vi "harp convert to csv.vi"() -> ()   [LabVIEW 2010]
uses:
  <vilib>/Utility/sysdir.llb/System Directory Type.ctl
panel:
  in  "error":string
  in  "don't\nask":bool
  in  "dummy 2":dbl caption="Available hidden commands:\nbootloader\ncreatecode\nresetcounters\nhardware"
  in  "ShowList":bool
  out "CameraBitPosition":i32
  out "Files to convert to CSV: 2":string
  in  "Match pattern: 2":string
  in  "Include subfolders: 2":bool=TRUE
  out "Overall progress: 2":dbl(slide) scale=0.0..1.0
  in  "Path (folder) 2":path caption="Path"
  out "Binary Harp folder: 2":string
  out "File progress: 2":dbl(slide) scale=0.0..1.0
  in  "Overwrite .csv files: 2":bool=TRUE
  in  "File extension: 2":string=".bin"
  in  "Execute parse on computer's RAM (faster): 2":bool=TRUE
  in  "System 2":bool
  in  "Create \"read me\" information file: 2":bool=TRUE
  in  "Filter: 2":T1(ring)
  in  "List: 2":string
  in  "Read 2":bool=TRUE
  in  "Write 2":bool=TRUE
  in  "Event 2":bool=TRUE
  in  "Save only if no error: 2":bool=TRUE
  in  "Round time to 4th decimal place: 2":bool=TRUE
  in  "Include entire information: 2":bool
  in  "Insert Bit Demux Elements at the end: 2":bool
  in  "For separation, use Tab instead of Comma:":bool
  out "System (copy)":bool
  in  "abort":bool
  out "conversion\ntime":u32
  in  "dummy":dbl
  out "Error Ctrl":bool
  in  "Create file with metadata information:":bool=TRUE
  in  "Show options":bool
  in  "Tab Control":T2(tab)
  in  "Tips":bool
  in  "Path (file)":path caption="Path"
  out "(1) Binary Harp file:":string
  in  "Convert":bool
  out "Progress:":dbl(slide) scale=0.0..1.0
  in  "Tips":bool
  out "Files to convert to CSV:":string="\r\n"
  in  "(14) Match pattern:":string
  in  "(12) Include subfolders:":bool=TRUE
  out "Overall progress:":dbl(slide) scale=0.0..1.0
  in  "Path (folder)":path caption="Path"
  out "(10) Binary Harp folder:":string
  in  "Convert 2":bool
  out "File progress:":dbl(slide) scale=0.0..1.0
  in  "(11) Overwrite .csv files:":bool=TRUE
  in  "(13) File extension:":string=".bin"
  in  "(41) Execute parse on computer's RAM (faster):":bool
  in  "System":bool
  in  "(30) Create \"read me\" information file:":bool=TRUE
  in  "(39) Filter:":T3(ring)
  in  "(40) List:":string caption="Separate the registers with a comma.\nExample: 8,32,33"
  in  "(32) Read":bool
  in  "(33) Write":bool
  in  "(34) Event":bool=TRUE
  in  "(35) Save only if no error:":bool=TRUE
  in  "(36) Round time to 4th decimal place:":bool=TRUE
  in  "(38) Include entire information:":bool
  in  "(37) Insert Bit Demux Elements at the end:":bool
  in  "Add register":bool
  in  "Quit":bool
  in  "Minimize":bool
  in  "Cam Tip":bool
  in  "Progress:":dbl(slide) scale=0.0..1.1
  in  "Convert 3":bool
  out "(60) Binary Harp file:":string
  in  "harp .bin":path caption="Path"
  out "(61) Camera metadata .csv file :":string
  in  "cam .csv":path caption="Path"
  in  "(62) Use Harp converted .csv file\nto timestamp the file:":bool=TRUE
  in  "Select Register":bool
  out "Pin name on the board:":string
  out "Raw Register Name:":string
  out "(64) Register Address:":i32
  in  "(63) Camera brand:":u16(ring) items=["PointGrey"]
  in  "EnableList":T4={"Cmd"=TRUE, "RegAdd"=TRUE, "Port"=FALSE, "Rsvd"=FALSE, "UTC"=TRUE, "Error"=FALSE, "Type"=FALSE, "NElements"=FALSE, "BitElementsColumn"=FALSE, "BitElementsAtTheEnd"=FALSE, "Read"=FALSE, "Write"=FALSE, "Event"=TRUE, "No Errors"=TRUE}
  # "Convert to CSV v1.9.0\nHardware Platform"
  # "Fractional number separation:"
  # "Separate the registers with a comma.\nExample: 8,32,33"
  # "Commands:"
  # "New columns will be added to the file\n(Port, Reserved, Error, Type and NumberOfElements)."
  # "The files with this pattern on the\nfile name will be converted to CSV.\nYou can leave it blank to select\nall files."
  # "Select the Harp binary file:"
  # "Select the folder where the Harp binary files exist:"
  # "The files with this pattern on the\nfile name will be converted to CSV.\nYou can leave it blank to select\nall files."
  # "Configuration of output files:"
  # "(31) Fractional number separation:"
  # "Commands:"
  # "New columns will be added to the file\n(Port, Reserved, Error, Type and NumberOfElements)."
  # "Select the files and the register:"
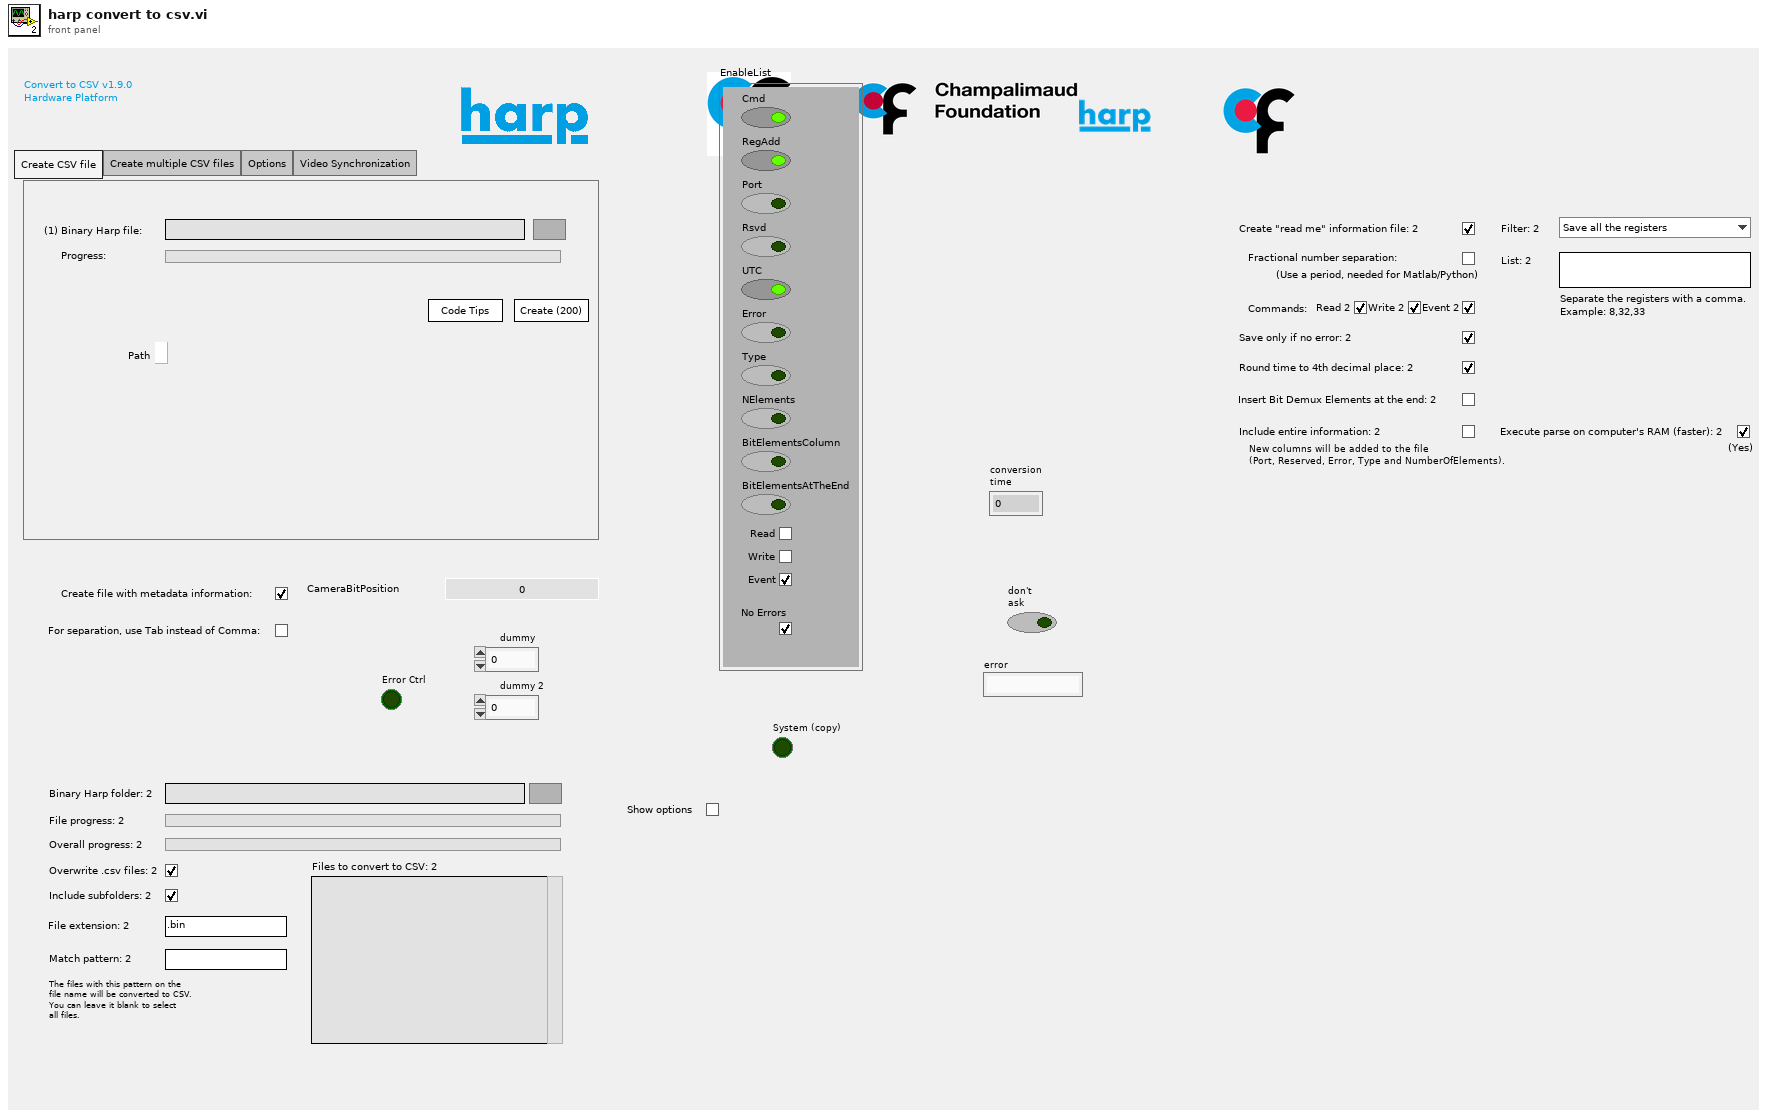
[diagram p1: front panel]
types:
  T1 = enum16{"Save all the registers", "Save only specific registers"}
  T2 = enum32{"Create CSV file", "Create multiple CSV files", "Options", "Video Synchronization"}
  T3 = enum16{"Save all the registers (0)", "Save only specific registers (1)"}
  T4 = cluster{"Cmd":bool, "RegAdd":bool, "Port":bool, "Rsvd":bool, "UTC":bool, "Error":bool, "Type":bool, "NElements":bool, "BitElementsColumn":bool, "BitElementsAtTheEnd":bool, "Read":bool, "Write":bool, "Event":bool, "No Errors":bool}
  T5 = enum32{"Invalid", "Standard", "Closed", "Hidden", "Minimized", "Maximized"}
  T6 = enum16{"Reset", "Get command", "Open files", "Freeze", "Unfreeze"}
  T7 = typedef "System Directory Type.ctl" = i32
  T8 = enum16{"open", "replace", "create", "open or create", "replace or create", "replace or create with confirmation"}
  T9 = enum32{"Create CSV file", "Create multiple CSV files", "Options"}
  T10 = enum8{"Enabled", "Disabled", "Disabled and Grayed Out"}
  T11 = cluster{"Create \"read me\" information file:":bool, "Create \"read me\" information file:":bool, "Create \"read me\" information file:":bool, "Create \"read me\" information file:":bool, "Create \"read me\" information file:":bool, "Create \"read me\" information file:":bool, "Create \"read me\" information file:":bool, "Create \"read me\" information file:":bool, "Create \"read me\" information file:":bool, "Filter:":enum16{"Save all the registers (0)", "Save only specific registers (1)"}, "List:":string, "Create \"read me\" information file:":bool, "List:":string, "List:":string, "Create \"read me\" information file:":bool, "Create \"read me\" information file:":bool, "List:":string, "List:":string, "List:":string, "List:":string, "Create \"read me\" information file:":bool, "List:":string, "RegisterAddress":i32, "List:":string, "RegisterAddress":i32}
  T12 = enum16{"Reset", "Get command", "Open files", "Freeze", "Unfreeze", "Save error"}
  T13 = enum16{"CreateBuffer", "WriteBytes", "WriteByte", "AvailableMemory", "OccupiedMemory", "CheckBytes", "ReadBytes"}
  T14 = cluster{"Device":string, "RegisterName":string, "PinBoardName":string, "CameraBitPosition":i32, "RegisterDescription":string, "IsUsedForCamera":bool, "RegisterAddress":i32, "RegisterRawName":string, "RegisterByteSize":i32}
  T15 = cluster{"(30) Create \"read me\" information file:":bool, "System":bool, "(32) Read":bool, "(33) Write":bool, "(34) Event":bool, "(35) Save only if no error:":bool, "(36) Round time to 4th decimal place:":bool, "(37) Insert Bit Demux Elements at the end:":bool, "(38) Include entire information:":bool, "(39) Filter:":enum16{"Save all the registers (0)", "Save only specific registers (1)"}, "(40) List:":string, "(41) Execute parse on computer's RAM (faster):":bool, "(1) Binary Harp file:":string, "(10) Binary Harp folder:":string, "(11) Overwrite .csv files:":bool, "(12) Include subfolders:":bool, "(13) File extension:":string, "(14) Match pattern:":string, "(60) Binary Harp file:":string, "(61) Camera metadata .csv file :":string, "(62) Use Harp converted .csv file\nto timestamp the file:":bool, "Raw Register Name:":string, "(64) Register Address:":i32, "Pin name on the board:":string, "CameraBitPosition":i32}
  T16 = cluster{"Timestamp(us)":dbl, "Command":u8, "Error":bool, "Register Address":u8, "Port":u8, "Number of Elements":u8, "Type":u8, "I8":i8, "U8":u8, "U16":u16, "I16":i16, "U32":u32, "I32":i32, "U64":u64, "I64":i64, "Float":sgl, "U8[]":u8[], "I8[]":i8[], "U16[]":u16[], "I16[]":i16[], "U32[]":u32[], "I32[]":i32[], "U64[]":u64[], "I64[]":i64[], "Float[]":sgl[]}
  T17 = enum16{"Left Button", "Center Button", "Right Button", "Window Close"}
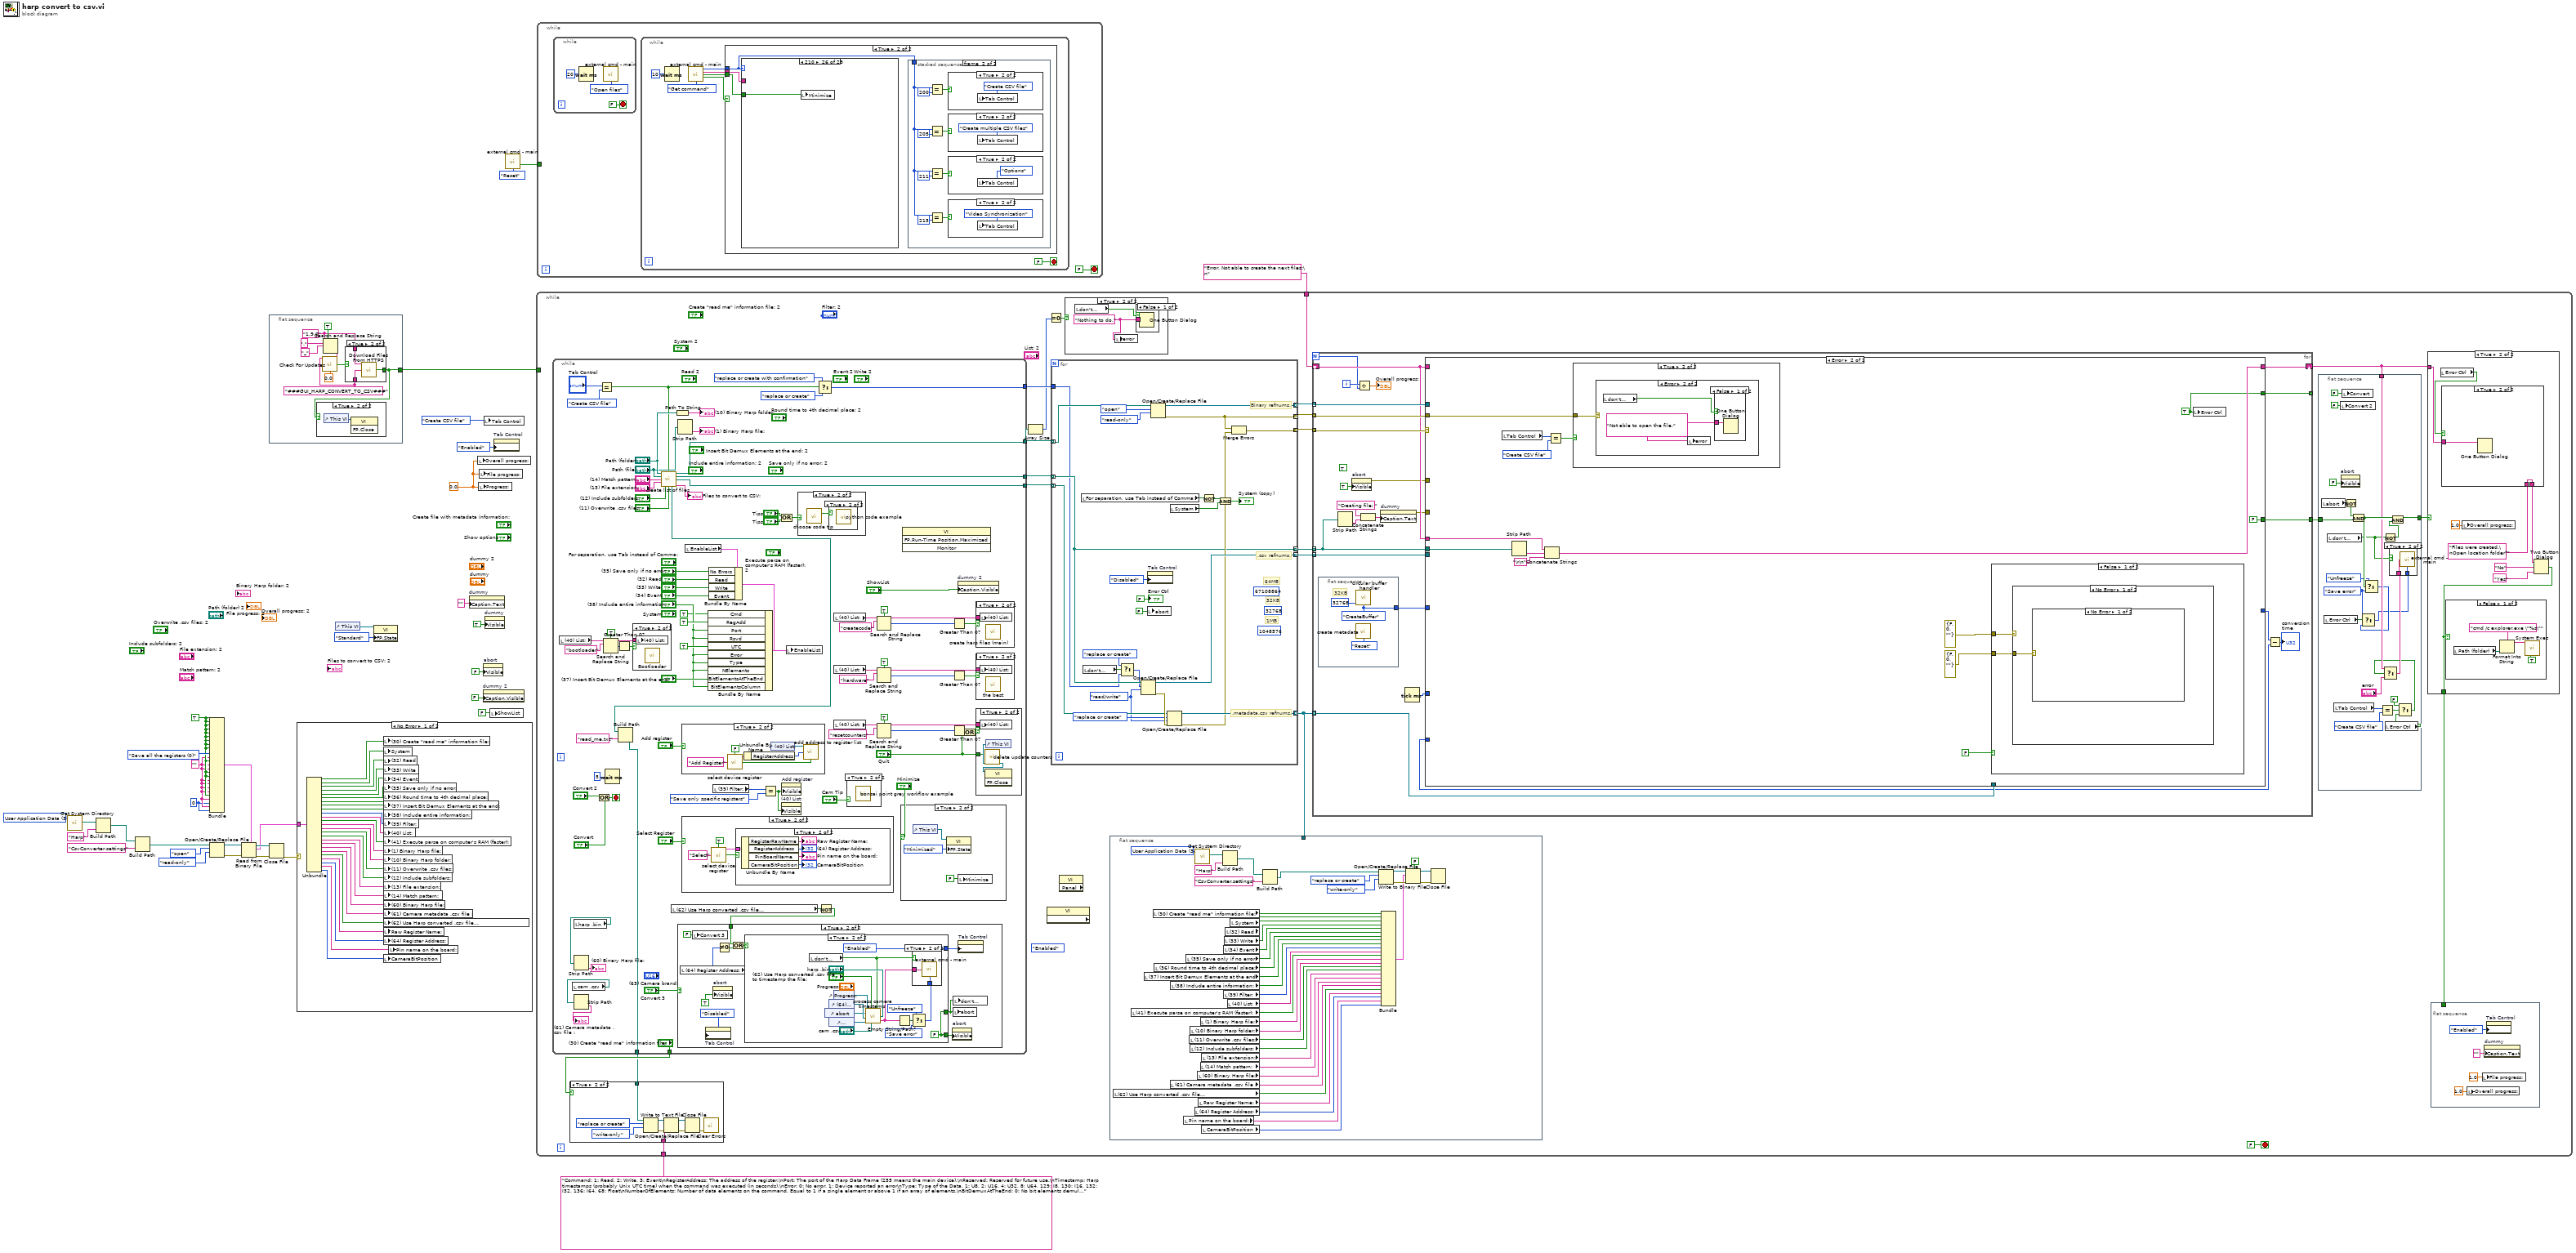
[diagram p0: block diagram]
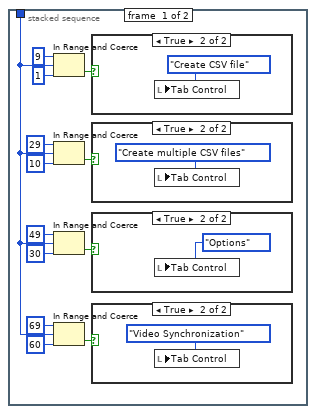
[diagram p3: hidden frame]
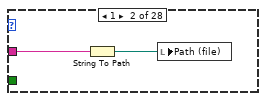
[diagram p13: hidden frame]
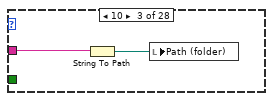
[diagram p14: hidden frame]
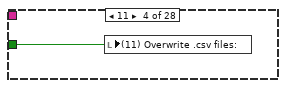
[diagram p15: hidden frame]
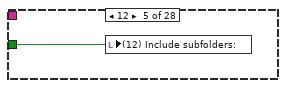
[diagram p16: hidden frame]
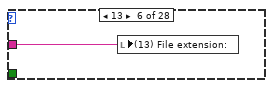
[diagram p17: hidden frame]
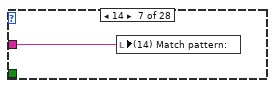
[diagram p18: hidden frame]
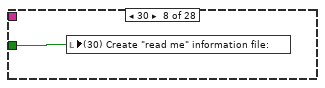
[diagram p19: hidden frame]
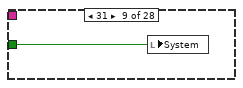
[diagram p20: hidden frame]
diagram:
  w6 = T7 3 items=["User Home"=0, "User Desktop"=1, "User Documents"=2, "User Application Data"=3, "User Preferences"=4, "User Temporary"=5, "Public Documents"=6, "Public Application Data"=7, "Public Preferences"=8, "Public Cache"=13, "System Core Libraries"=9, "System Installed Libraries"=10, "Application Files"=11, "Boot Volume Root"=12] ("system directory type")
  w9 = 0 ("RegisterAddress")
  w10 = "" ("List:")
  w11 = TRUE ("Create \"read me\" information file:")
  w32 = 0.0 ("Processing")
  n1 = call <vilib>:"Get System Directory.vi"("system directory type"=w6) -> ("system directory"=w7:path)  [unwired: 10 in]
  n2 = Build Path(base path=w7, name or relative path="Harp") -> (appended path=w5:path)
  n3 = Build Path(base path=w5, name or relative path="CsvConverter.settings") -> (appended path=w12:path)
  n4 = Bundle("Create \"read me\" information file:"=w11, "Create \"read me\" information file:"=w11, "Create \"read me\" information file:"=w11, "Create \"read me\" information file:"=w11, "Create \"read me\" information file:"=w11, "Create \"read me\" information file:"=w11, "Create \"read me\" information file:"=w11, "Create \"read me\" information file:"=w11, "Create \"read me\" information file:"=w11, "Filter:"=T3."Save all the registers (0)", "List:"=w10, "Create \"read me\" information file:"=w11, "List:"=w10, "List:"=w10, "Create \"read me\" information file:"=w11, "Create \"read me\" information file:"=w11, "List:"=w10, "List:"=w10, "List:"=w10, "List:"=w10, "Create \"read me\" information file:"=w11, "List:"=w10, "RegisterAddress"=w9, "List:"=w10, "RegisterAddress"=w9) -> (w19:T11)  [unwired: 1 in]
  n5 = Open/Create/Replace File(file path (use dialog)=w12, operation (0:open)=T8."open", access (0:read/write)=enum16{"read/write", "read-only", "write-only"}."read-only") -> (refnum out=w17:refnum<file>, error out=w16:errorcluster)  [unwired: 3 in, 1 out]
  n6 = Read from Binary File(5:w19, 8:w16, 11:w17) -> (0:w21:errorcluster, 2:w20:T11, 3:w22:refnum<file>)  [unwired: 3 in, 1 out]
  n7 = flat-sequence {
    tunnel: [w36] -> w26
    frame #0 {
      w39 = "1.9.0" ("current version")
      w38 = "###GUI_HARP_CONVERT_TO_CSV###" ("name or relative path")
      n8 = Search and Replace String(replace all?=TRUE ("replace all? (F)"), input string=w39, search string=".", replace string="_" ("replace string (\"\")")) -> (result string=w40:string)  [unwired: 4 in, 3 out]
      n9 = call "Check For Updates.vi"("GUI search key"=w38, "shortcut key"=w40, "timeout (days)"=0.0) -> ("check for updates"=w37:bool)  [unwired: 12 in]
      n10 = case shown="True" w37 {
        tunnel: w38 -> [_ w48]
        tunnel: w39 -> [_ w47]
        tunnel: [FALSE ("updated") w46] -> w36
        frame False {
        }
        frame True {
          n11 = call "Download Files From HTTPS.vi"("current version"=w47, "GUI search key"=w48) -> ("updated"=w46:bool)  [unwired: 13 in]
        }
      }
      n12 = case shown="True" w36 {
        frame False {
        }
        frame True {
          n13 = control-ref of="This VI"() -> (w44:refnum<vi>)
          n14 = invoke class="VI" method="FP.Close"(reference=w44) -> ()  [unwired: 2 in, 3 out]
        }
      }
    }
  }
  n15 = Close File(refnum=w22, error in=w21) -> (error out=w23:errorcluster)  [unwired: 1 out]
  n16 = case shown="No Error" w23 {
    tunnel: w20 -> [w74 _]
    frame No Error {
      n17 = Unbundle(w74) -> ("Create \"read me\" information file:"=w73:bool, "Create \"read me\" information file:"=w72:bool, "Create \"read me\" information file:"=w71:bool, "Create \"read me\" information file:"=w70:bool, "Create \"read me\" information file:"=w69:bool, "Create \"read me\" information file:"=w68:bool, "Create \"read me\" information file:"=w67:bool, "Create \"read me\" information file:"=w66:bool, "Create \"read me\" information file:"=w65:bool, "Filter:"=w64:T3, "List:"=w63:string, "Create \"read me\" information file:"=w62:bool, "List:"=w61:string, "List:"=w60:string, "Create \"read me\" information file:"=w59:bool, "Create \"read me\" information file:"=w58:bool, "List:"=w57:string, "List:"=w56:string, "List:"=w55:string, "List:"=w54:string, "Create \"read me\" information file:"=w53:bool, "List:"=w52:string, "RegisterAddress"=w51:i32, "List:"=w50:string, "RegisterAddress"=w49:i32)
      n18 = local write "(30) Create \"read me\" information file:"(w73) -> ()
      n19 = local write "System"(w72) -> ()
      n20 = local write "(32) Read"(w71) -> ()
      n21 = local write "(33) Write"(w70) -> ()
      n22 = local write "(34) Event"(w69) -> ()
      n23 = local write "(35) Save only if no error:"(w68) -> ()
      n24 = local write "(36) Round time to 4th decimal place:"(w67) -> ()
      n25 = local write "(37) Insert Bit Demux Elements at the end:"(w66) -> ()
      n26 = local write "(38) Include entire information:"(w65) -> ()
      n27 = local write "(39) Filter:"(w64) -> ()
      n28 = local write "(40) List:"(w63) -> ()
      n29 = local write "(41) Execute parse on computer's RAM (faster):"(w62) -> ()
      n30 = local write "(1) Binary Harp file:"(w61) -> ()
      n31 = local write "(10) Binary Harp folder:"(w60) -> ()
      n32 = local write "(11) Overwrite .csv files:"(w59) -> ()
      n33 = local write "(12) Include subfolders:"(w58) -> ()
      n34 = local write "(13) File extension:"(w57) -> ()
      n35 = local write "(14) Match pattern:"(w56) -> ()
      n36 = local write "(60) Binary Harp file:"(w55) -> ()
      n37 = local write "(61) Camera metadata .csv file :"(w54) -> ()
      n38 = local write "(62) Use Harp converted .csv file\nto timestamp the file:"(w53) -> ()
      n39 = local write "Raw Register Name:"(w52) -> ()
      n40 = local write "(64) Register Address:"(w51) -> ()
      n41 = local write "CameraBitPosition"(w49) -> ()
      n42 = local write "Pin name on the board:"(w50) -> ()
    }
    frame Error {
    }
  }
  n43 = control-ref of="This VI"() -> (w1:refnum<vi>)
  n44 = property class="VI"(reference=w1, "FP.State"=T5."Standard" ("Front Panel Window:State")) -> ()  [unwired: 1 in, 2 out]
  n45 = property on="dummy" class="DigNum (strict)"("Caption.Text"="") -> ()  [unwired: 2 in, 2 out]
  n46 = local write "Overall progress:"(w32) -> ()
  n47 = local write "Progress:"(w32) -> ()
  n48 = local write "File progress:"(w32) -> ()
  n49 = property on="dummy 2" class="DigNum (strict)"("Caption.Visible"=FALSE) -> ()  [unwired: 2 in, 2 out]
  n50 = property on="abort" class="Bool (strict)"("Visible"=FALSE) -> ()  [unwired: 2 in, 2 out]
  n51 = local write "Tab Control"(T9."Create CSV file" ("y")) -> ()
  n52 = property on="dummy" class="DigNum (strict)"("Visible"=TRUE) -> ()  [unwired: 2 in, 2 out]
  n53 = local write "ShowList"(FALSE ("ShowList")) -> ()
  n54 = property on="Tab Control" class="TabCtl (strict)"("DisabledEnum"=T10."Enabled" ("Disabled")) -> ()  [unwired: 2 in, 2 out]
  n55 = call "external cmd - main.vi"("option"=T6."Reset") -> ("cmd available"=w4:bool)  [unwired: 11 in, 3 out]
  n56 = while {
    tunnel: "Command: 1: Read, 2: Write, 3: Event\nRegisterAddress: The address of the register.\nPort: The port of the Harp Data Frame (255 means the main device).\nReserved: Reserved for future use.\nTimestamp: Harp timestamps (probably Unix UTC time) when the command was executed (in seconds).\nError: 0: No error, 1: Device reported an error\nType: Type of the Data. 1: U8, 2: U16, 4: U32, 8: U64, 129: I8, 130: I16, 132: I32, 136: I64, 68: Float\nNumberOfElements: Number of data elements on the command. Equal to 1 if a single element or above 1 if an array of elements.\nBitDemuxAtTheEnd: 0: No bit elements demultiplexer on the end of the command line, 1: Bit elements and the end (always 1 when it's a single element)\nDataElement0: First data element of the command (unique if the command has only a single element)." ("string") -> [w91]
    tunnel: "Error. Not able to create the next files:\n" -> [w85]
    tunnel: w26 -> [_]
    stop <- FALSE stop-if-true
    (unwired) T10."Enabled" ("Disabled")
    n57 = while {
      tunnel: ["(30) Create \"read me\" information file:"] -> w92
      tunnel: [w512] -> w90
      tunnel: [w498] -> w78
      tunnel: [w497] -> w89
      tunnel: [w496] -> w80
      tunnel: [w492] -> w88
      stop <- w488 stop-if-true
      n58 = local read "(40) List:"() -> (w480:string)
      n59 = local read "cam .csv"() -> (w467:path)
      n60 = local read "harp .bin"() -> (w469:path)
      n61 = Strip Path(path=w469) -> (name=→"(60) Binary Harp file:":string)  [unwired: 1 out]
      n62 = Strip Path(path=w467) -> (name=→"(61) Camera metadata .csv file :":string)  [unwired: 1 out]
      n63 = Or(x="Convert 2", y="Convert") -> (x .or. y?=w488:bool)
      n64 = Equal?(x="Tab Control", y=T9."Create CSV file") -> (x = y?=w495:bool)
      n65 = Search and Replace String(case sensitive?=TRUE ("ignore case? (F)"), input string=w480, search string="bootloader") -> (result string=w476:string, number of replacements=w478:i32)  [unwired: 5 in, 2 out]
      n66 = Wait (ms)(milliseconds to wait=u32 5) -> ()  [unwired: 1 out]
      n67 = Greater Than 0?(x=w478) -> (x > 0?=w477:bool)
      n68 = case shown="True" w477 {
        tunnel: w476 -> [_ w581]
        frame False {
        }
        frame True {
          n69 = local write "(40) List:"(w581) -> ()
          n70 = call "Bootloader.vi"() -> ()  [unwired: 12 in]
        }
      }
      n71 = call "create list of files.vi"("Path (folder) 2"="Path (folder)", "Single file (T)"=w495, "Path (file)"="Path (file)", "Match pattern:"="(14) Match pattern:", "File extension:"="(13) File extension:", "Subfolders?"="(12) Include subfolders:", "Overwrite .csv files:"="(11) Overwrite .csv files:") -> ("Array of files to be converted"=w498:path[], "Array of .csv"=w497:path[], "Array of .metadat.csv"=w496:path[], "Path for read me"=w491:path, "Files to convert to CSV:"=→"Files to convert to CSV:":string)  [unwired: 4 in]
      n72 = Build Path(base path=w491, name or relative path="read_me.txt") -> (appended path=w512:path)
      n73 = local read "(62) Use Harp converted .csv file\nto timestamp the file:"() -> (w465:bool)
      n74 = Path To String(path="Path (folder)") -> (string=→"(10) Binary Harp folder:":string)
      n75 = Strip Path(path="Path (file)") -> (name=→"(1) Binary Harp file:":string)  [unwired: 1 out]
      n76 = case shown="True" "Add register" {
        frame False {
        }
        frame True {
          n77 = call "select device register.vi"("Camera registers (T) / All Registers (F)"=FALSE, "Ok Button"="Add Register") -> ("Selected Register"=w579:T14, "Register Selected"=w576:bool)  [unwired: 12 in]
          n78 = Unbundle By Name(w579) -> ("RegisterAddress"=w577:i32)
          n79 = control-ref of="(40) List:"() -> (w578:refnum<vi>)
          n80 = call "add address to register list.vi"("reference"=w578, "RegisterAddress"=w577, "Register Selected"=w576) -> ()  [unwired: 13 in]
        }
      }
      n81 = case shown="True" "Select Register" {
        frame False {
        }
        frame True {
          n82 = call "select device register.vi"("Camera registers (T) / All Registers (F)"=TRUE, "Ok Button"="Select") -> ("Selected Register"=w567:T14, "Register Selected"=w566:bool)  [unwired: 12 in]
          n83 = case shown="True" w566 {
            tunnel: w567 -> [_ w574]
            frame False {
            }
            frame True {
              n84 = Unbundle By Name(w574) -> ("RegisterRawName"=→"Raw Register Name:":string, "RegisterAddress"=→"(64) Register Address:":i32, "PinBoardName"=→"Pin name on the board:":string, "CameraBitPosition"=→"CameraBitPosition":i32)
            }
          }
        }
      }
      n85 = local read "EnableList"() -> (w519:T4)
      n86 = Bundle By Name(cluster=w519, "No Errors"="(35) Save only if no error:", "Read"="(32) Read", "Write"="(33) Write", "Event"="(34) Event") -> (w514:T4)
      n87 = Bundle By Name(cluster=w514, "Cmd"=TRUE, "RegAdd"=TRUE, "Port"="(38) Include entire information:", "Rsvd"="(38) Include entire information:", "UTC"=TRUE, "Error"="(38) Include entire information:", "Type"="(38) Include entire information:", "NElements"="(38) Include entire information:", "BitElementsAtTheEnd"="(37) Insert Bit Demux Elements at the end:", "BitElementsColumn"="(38) Include entire information:") -> (w521:T4)
      n88 = local read "(39) Filter:"() -> (w475:T3)
      n89 = Equal?(x=w475, y=T1."Save only specific registers") -> (x = y?=w442:bool)
      n90 = Or(x="Tips", y="Tips") -> (x .or. y?=w482:bool)
      n91 = property on="(40) List:" class="Str"("Visible"=w442) -> ()  [unwired: 2 in, 2 out]
      n92 = property on="Add register" class="Bool"("Visible"=w442) -> ()  [unwired: 2 in, 2 out]
      n93 = local write "EnableList"(w521) -> ()
      n94 = case shown="True" w482 {
        frame False {
        }
        frame True {
          n95 = call "choose code tip.vi"() -> ("Python"=w582:bool)  [unwired: 14 in, 1 out]
          n96 = case shown="True" w582 {
            frame False {
              n97 = call "matlab code example.vi"() -> ()  [unwired: 12 in]
            }
            frame True {
              n98 = call "python code example.vi"() -> ()  [unwired: 12 in]
            }
          }
        }
      }
      n99 = Select(t=T8."replace or create with confirmation" ("operation (0:open)"), s=w495, f=T8."replace or create" ("operation (0:open)")) -> (s? t:f=w492:T8)
      n100 = Not(x=w465) -> (.not. x?=w464:bool)
      n101 = case shown="True" "Convert 3" {
        tunnel: w464 -> [_ w539]
        frame False {
        }
        frame True {
          n102 = local read "(64) Register Address:"() -> (w532:i32)
          n103 = local write "Convert 3"(FALSE ("Convert 3")) -> ()
          n104 = property on="Tab Control" class="TabCtl (strict)"("DisabledEnum"=T10."Disabled" ("Disabled")) -> ()  [unwired: 2 in, 2 out]
          n105 = property on="abort" class="Bool (strict)"("Visible"=TRUE) -> ()  [unwired: 2 in, 2 out]
          n106 = Not Equal To 0?(x=w532) -> (x != 0?=w541:bool)
          n107 = Or(x=w539, y=w541) -> (x .or. y?=w540:bool)
          n108 = case shown="True" w540 {
            tunnel: [w544 w556] -> w537
            tunnel: [w544 w556] -> w533
            tunnel: [T10."Enabled" ("Disabled") T10."Enabled" ("Disabled")] -> w535
            frame False {
              w544 = FALSE ("Visible")
              n109 = local read "don't\nask"() -> (w542:bool)
              n110 = case shown="False" w542 {
                tunnel: "Error. Register was not selected." ("message") -> [w546 w548]
                frame False {
                  n111 = One Button Dialog(message=w546) -> ()  [unwired: 1 in, 1 out]
                }
                frame True {
                  n112 = call "external cmd - main.vi"("error"=w548, "option"=T12."Save error") -> ()  [unwired: 10 in, 4 out]
                }
              }
            }
            frame True {
              w556 = FALSE ("Visible")
              n113 = local read "don't\nask"() -> (w549:bool)
              n114 = control-ref of="abort"() -> (w561:refnum<vi>)
              n115 = control-ref of="(64) Register Address:"() -> (w562:refnum<vi>)
              n116 = control-ref of="CameraBitPosition"() -> (w563:refnum<vi>)
              n117 = control-ref of="Progress:"() -> (w560:refnum<vi>)
              n118 = call "process camera timestamp.vi"("Progress:"=w560, "Use Harp converted .csv file\nto timestamp the file:"="(62) Use Harp converted .csv file\nto timestamp the file:", "abort"=w561, "Register Address:"=w562, "cam .csv"="cam .csv", "CameraBitPosition"=w563, "don't ask"=w549, "harp .bin"="harp .bin") -> ("error"=w550:string)
              n119 = Empty String/Path?(string/path=w550) -> (empty?=w554:bool)
              n120 = Select(t=T12."Unfreeze" ("option"), s=w554, f=T12."Save error" ("option")) -> (s? t:f=w551:T12)
              n121 = case shown="True" w549 {
                tunnel: w551 -> [_ w565]
                tunnel: w550 -> [_ w564]
                frame False {
                }
                frame True {
                  n122 = call "external cmd - main.vi"("error"=w564, "option"=w565) -> ()  [unwired: 10 in, 4 out]
                }
              }
            }
          }
          n123 = property on="abort" class="Bool (strict)"("Visible"=w537) -> ()  [unwired: 2 in, 2 out]
          n124 = local write "abort"(w533) -> ()
          n125 = local write "don't\nask"(w533) -> ()
          n126 = property on="Tab Control" class="TabCtl (strict)"("DisabledEnum"=w535) -> ()  [unwired: 2 in, 2 out]
        }
      }
      n127 = local read "(40) List:"() -> (w459:string)
      n128 = local read "(40) List:"() -> (w456:string)
      n129 = local read "(40) List:"() -> (w447:string)
      n130 = case shown="True" "Cam Tip" {
        frame False {
        }
        frame True {
          n131 = call "bonsai point grey workflow example.vi"() -> ()  [unwired: 12 in]
        }
      }
      n132 = Search and Replace String(case sensitive?=TRUE ("ignore case? (F)"), input string=w459, search string="createcode") -> (result string=w463:string, number of replacements=w461:i32)  [unwired: 5 in, 2 out]
      n133 = Search and Replace String(case sensitive?=TRUE ("ignore case? (F)"), input string=w456, search string="hardware") -> (result string=w452:string, number of replacements=w454:i32)  [unwired: 5 in, 2 out]
      n134 = Search and Replace String(case sensitive?=TRUE ("ignore case? (F)"), input string=w447, search string="resetcounters") -> (result string=w451:string, number of replacements=w449:i32)  [unwired: 5 in, 2 out]
      n135 = case shown="True" "Minimize" {
        frame False {
        }
        frame True {
          n136 = control-ref of="This VI"() -> (w523:refnum<vi>)
          n137 = property class="VI"(reference=w523, "FP.State"=T5."Minimized" ("Front Panel Window:State")) -> ()  [unwired: 1 in, 2 out]
          n138 = local write "Minimize"(FALSE ("Minimize")) -> ()
        }
      }
      n139 = invoke class="VI" method="FP.Run-Time Position.Maximized"() -> ()  [unwired: 4 in, 4 out]
      n140 = Greater Than 0?(x=w461) -> (x > 0?=w462:bool)
      n141 = Greater Than 0?(x=w454) -> (x > 0?=w453:bool)
      n142 = Greater Than 0?(x=w449) -> (x > 0?=w450:bool)
      n143 = property on="dummy 2" class="DigNum (strict)"("Caption.Visible"="ShowList") -> ()  [unwired: 2 in, 2 out]
      n144 = Or(x=w450, y="Quit") -> (x .or. y?=w444:bool)
      n145 = case shown="True" w462 {
        tunnel: w463 -> [_ w531]
        frame False {
        }
        frame True {
          n146 = local write "(40) List:"(w531) -> ()
          n147 = call "create harp files (main).vi"() -> ()  [unwired: 12 in]
        }
      }
      n148 = case shown="True" w453 {
        tunnel: w452 -> [_ w530]
        frame False {
        }
        frame True {
          n149 = local write "(40) List:"(w530) -> ()
          n150 = call "the best.vi"() -> ()  [unwired: 12 in]
        }
      }
      n151 = case shown="True" w444 {
        tunnel: w451 -> [_ w529]
        tunnel: "Quit" -> [_ w526]
        frame False {
        }
        frame True {
          n152 = local write "(40) List:"(w529) -> ()
          n153 = control-ref of="This VI"() -> (w528:refnum<vi>)
          n154 = call "delete update counters.vi"("This VI"=w528, "just quit"=w526) -> ("This VI"=w527:refnum<vi>)  [unwired: 9 in]
          n155 = invoke class="VI" method="FP.Close"(reference=w527) -> ()  [unwired: 2 in, 3 out]
        }
      }
    }
    n156 = case shown="True" w92 {
      tunnel: w91 -> [_ w435]
      tunnel: w90 -> [_ w434]
      frame False {
      }
      frame True {
        n157 = Open/Create/Replace File(file path (use dialog)=w434, operation (0:open)=T8."replace or create", access (0:read/write)=enum16{"read/write", "read-only", "write-only"}."write-only") -> (refnum out=w432:refnum<file>, error out=w438:errorcluster)  [unwired: 3 in, 1 out]
        n158 = Write to Text File(file (use dialog)=w432, text=w435, error in=w438) -> (refnum out=w433:refnum<file>, error out=w439:errorcluster)  [unwired: 1 in, 1 out]
        n159 = Close File(refnum=w433, error in=w439) -> (error out=w440:errorcluster)  [unwired: 1 out]
        n160 = call <vilib>:"Clear Errors.vi"("error in (no error)"=w440) -> ()  [unwired: 6 in, 1 out]
      }
    }
    n161 = Array Size(array=w78) -> (size(s)=w77:i32)
    n162 = property class="VI" props=["Front Panel.Minimizeable"]() -> ()  [unwired: 2 in, 3 out]
    n163 = Equal To 0?(x=w77) -> (x = 0?=w79:bool)
    n164 = for {
      tunnel: [w431] -> w95 mode=indexing
      tunnel: [w430] -> w87 mode=indexing
      tunnel: [w429] -> w94 mode=indexing
      tunnel: w78 -> [w426] mode=indexing
      tunnel: w89 -> [w418] mode=indexing
      tunnel: w80 -> [w424] mode=indexing
      tunnel: w88 -> [w409]
      tunnel: [w421] -> w76 mode=indexing
      tunnel: [w420] -> w86 mode=indexing
      tunnel: [w418] -> w84 mode=indexing
      (unwired) 1048576 ("NumberOfBytes")
      (unwired) 67108864 ("NumberOfBytes")
      (unwired) 32768 ("NumberOfBytes")
      w422 = enum16{"read/write", "read-only", "write-only"}."read/write" ("access (0:read/write)")
      # "1MB"
      # "64MB"
      # "32KB"
      # ".metadata.csv refnums."
      # ".csv refnums."
      # "Binary refnums."
      n165 = local read "For separation, use Tab instead of Comma:"() -> (w414:bool)
      n166 = local read "don't\nask"() -> (w410:bool)
      n167 = Select(t=T8."replace or create" ("operation (0:open)"), s=w410, f=w409) -> (s? t:f=w408:T8)
      n168 = Open/Create/Replace File(file path (use dialog)=w418, operation (0:open)=w408, access (0:read/write)=w422) -> (refnum out=w429:refnum<file>, error out=w425:errorcluster)  [unwired: 3 in, 1 out]
      n169 = local write "abort"(FALSE ("abort")) -> ()
      n170 = property on="Tab Control" class="TabCtl (strict)"("DisabledEnum"=T10."Disabled" ("Disabled")) -> ()  [unwired: 2 in, 2 out]
      n171 = Open/Create/Replace File(file path (use dialog)=w426, operation (0:open)=T8."open", access (0:read/write)=enum16{"read/write", "read-only", "write-only"}."read-only") -> (refnum out=w431:refnum<file>, error out=w420:errorcluster)  [unwired: 3 in, 1 out]
      n172 = Open/Create/Replace File(file path (use dialog)=w424, error in=w425, operation (0:open)=T8."replace or create", access (0:read/write)=w422) -> (refnum out=w421:refnum<file>, error out=w419:errorcluster)  [unwired: 2 in, 1 out]
      n173 = local read "System"() -> (w412:bool)
      n174 = Not(x=w414) -> (.not. x?=w413:bool)
      n175 = And(x=w413, y=w412) -> (x .and. y?=→"System (copy)":bool)
      n176 = Merge Errors(w420, w419) -> (w430:errorcluster)
      "Error Ctrl" <- FALSE ("Error Ctrl")
    }
    n177 = property class="VI" props=["Panel"]() -> ()  [unwired: 2 in, 3 out]
    n178 = case shown="True" w79 {
      frame False {
      }
      frame True {
        w135 = "Nothing to do." ("message")
        n179 = local read "don't\nask"() -> (w136:bool)
        n180 = local write "error"(w135) -> ()
        n181 = case shown="False" w136 {
          tunnel: w135 -> [w137 _]
          frame False {
            n182 = One Button Dialog(message=w137) -> ()  [unwired: 1 in, 1 out]
          }
          frame True {
          }
        }
      }
    }
    n183 = flat-sequence {
      tunnel: w76 -> [_]
      frame #0 {
        w98 = T7 3 items=["User Home"=0, "User Desktop"=1, "User Documents"=2, "User Application Data"=3, "User Preferences"=4, "User Temporary"=5, "Public Documents"=6, "Public Application Data"=7, "Public Preferences"=8, "Public Cache"=13, "System Core Libraries"=9, "System Installed Libraries"=10, "Application Files"=11, "Boot Volume Root"=12] ("system directory type")
        n184 = local read "(62) Use Harp converted .csv file\nto timestamp the file:"() -> (w106:bool)
        n185 = local read "(41) Execute parse on computer's RAM (faster):"() -> (w123:bool)
        n186 = local read "(37) Insert Bit Demux Elements at the end:"() -> (w127:bool)
        n187 = local read "(30) Create \"read me\" information file:"() -> (w134:bool)
        n188 = local read "(36) Round time to 4th decimal place:"() -> (w128:bool)
        n189 = local read "(61) Camera metadata .csv file :"() -> (w107:string)
        n190 = local read "(38) Include entire information:"() -> (w126:bool)
        n191 = local read "Pin name on the board:"() -> (w103:string)
        n192 = local read "(35) Save only if no error:"() -> (w129:bool)
        n193 = local read "(11) Overwrite .csv files:"() -> (w112:bool)
        n194 = local read "(12) Include subfolders:"() -> (w111:bool)
        n195 = local read "(10) Binary Harp folder:"() -> (w113:string)
        n196 = local read "(64) Register Address:"() -> (w104:i32)
        n197 = call <vilib>:"Get System Directory.vi"("system directory type"=w98) -> ("system directory"=w99:path)  [unwired: 10 in]
        n198 = local read "(60) Binary Harp file:"() -> (w108:string)
        n199 = local read "Raw Register Name:"() -> (w105:string)
        n200 = local read "(1) Binary Harp file:"() -> (w114:string)
        n201 = local read "(14) Match pattern:"() -> (w109:string)
        n202 = local read "(13) File extension:"() -> (w110:string)
        n203 = local read "CameraBitPosition"() -> (w102:i32)
        n204 = Build Path(base path=w99, name or relative path="Harp") -> (appended path=w97:path)
        n205 = local read "(34) Event"() -> (w130:bool)
        n206 = local read "(39) Filter:"() -> (w125:T3)
        n207 = local read "(33) Write"() -> (w131:bool)
        n208 = local read "(32) Read"() -> (w132:bool)
        n209 = local read "(40) List:"() -> (w124:string)
        n210 = local read "System"() -> (w133:bool)
        n211 = Build Path(base path=w97, name or relative path="CsvConverter.settings") -> (appended path=w96:path)
        n212 = Open/Create/Replace File(file path (use dialog)=w96, operation (0:open)=T8."replace or create", access (0:read/write)=enum16{"read/write", "read-only", "write-only"}."write-only") -> (refnum out=w120:refnum<file>, error out=w119:errorcluster)  [unwired: 3 in, 1 out]
        n213 = Bundle("(30) Create \"read me\" information file:"=w134, "System"=w133, "(32) Read"=w132, "(33) Write"=w131, "(34) Event"=w130, "(35) Save only if no error:"=w129, "(36) Round time to 4th decimal place:"=w128, "(37) Insert Bit Demux Elements at the end:"=w127, "(38) Include entire information:"=w126, "(39) Filter:"=w125, "(40) List:"=w124, "(41) Execute parse on computer's RAM (faster):"=w123, "(1) Binary Harp file:"=w114, "(10) Binary Harp folder:"=w113, "(11) Overwrite .csv files:"=w112, "(12) Include subfolders:"=w111, "(13) File extension:"=w110, "(14) Match pattern:"=w109, "(60) Binary Harp file:"=w108, "(61) Camera metadata .csv file :"=w107, "(62) Use Harp converted .csv file\nto timestamp the file:"=w106, "Raw Register Name:"=w105, "(64) Register Address:"=w104, "Pin name on the board:"=w103, "CameraBitPosition"=w102) -> (w115:T15)  [unwired: 1 in]
        n214 = Write to Binary File(file (use dialog)=w120, data=w115, error in=w119, 5:FALSE ("prepend array or string size? (T)")) -> (refnum out=w116:refnum<file>, error out=w117:errorcluster)  [unwired: 2 in, 1 out]
        n215 = Close File(refnum=w116, error in=w117) -> ()  [unwired: 2 out]
      }
    }
    n216 = for {
      N -> [w198]
      tunnel: w95 -> [w207] mode=indexing
      tunnel: w94 -> [w206] mode=indexing
      tunnel: w76 -> [w204] mode=indexing
      tunnel: w87 -> [w203] mode=indexing
      tunnel: w86 -> [w202] mode=indexing
      shift-right: [w201] -> w75
      shift-left: w85 -> [w200]
      tunnel: w84 -> [w191] mode=indexing
      tunnel: [w196] -> _ mode=indexing
      tunnel: [w195] -> w83
      i -> [w199]
      (unwired) TRUE ("Visible")
      n217 = flat-sequence {
        tunnel: [w209] -> w205
        frame #0 {
          w209 = T13."CreateBuffer" ("Enum")
          # "32KB"
          n218 = call "create metadata.vi"("Enum"=enum16{"Find Match", "Reset"}."Reset") -> ()  [unwired: 13 in, 2 out]
          n219 = call "circular buffer handler.vi"("NumberOfBytes"=32768, "Enum"=w209) -> ()  [unwired: 11 in, 3 out]
        }
      }
      n220 = Strip Path(path=w191) -> (name=w192:string)  [unwired: 1 out]
      n221 = property on="abort" class="Bool (strict)"("Visible"=TRUE) -> (error out=w184:errorcluster)  [unwired: 2 in, 1 out]
      n222 = Divide(x=w199, y=w198) -> (x/y=→"Overall progress:":dbl)
      n223 = Concatenate Strings("Creating file: " ("string"), w192) -> (w194:string)
      n224 = property on="dummy" class="DigNum (strict)"("Caption.Text"=w194) -> (error out=w190:errorcluster)  [unwired: 2 in, 1 out]
      n225 = Tick Count (ms)() -> (millisecond timer value=w188:u32)
      n226 = case shown="Error" w203 {
        tunnel: w207 -> [w225 _]
        tunnel: w206 -> [w230 _]
        tunnel: w205 -> [_ _]
        tunnel: w204 -> [w233 _]
        tunnel: w202 -> [_ w397]
        tunnel: w191 -> [_ w390]
        tunnel: w200 -> [_ w387]
        tunnel: [w223 w386] -> w201
        tunnel: w200 -> [w223 _]
        tunnel: [_ w385] -> w196
        tunnel: [w222 FALSE] -> w195
        tunnel: w190 -> [_ _]
        tunnel: [w217 _] -> w189
        tunnel: w188 -> [w216 _]
        tunnel: [w216 _] -> w187
        tunnel: w184 -> [_ _]
        frame No Error {
          (unwired) 262144 ("y")
          (unwired) 8096 ("y")
          w215 = ""
          # "256KB"
          # "8KB"
          # "Stop Criteria"
          n227 = local read "EnableList"() -> (w237:T4)
          n228 = local read "For separation, use Tab instead of Comma:"() -> (w211:bool)
          n229 = call "create header.vi"("Use Tab (T) ot Comma (F)"=w211, "EnableList"=w237) -> ("Line"=w231:string)  [unwired: 13 in]
          n230 = Get File Size(file=w225) -> (refnum out=w242:refnum<file>, size (in bytes)=w239:i64, 0:w241:errorcluster)  [unwired: 1 in]
          n231 = Write to Text File(file (use dialog)=w230, text=w231) -> (refnum out=w229:refnum<file>, error out=w232:errorcluster)  [unwired: 2 in, 1 out]
          n232 = call <vilib>:"Clear Errors.vi"("error in (no error)"=w241) -> ()  [unwired: 6 in, 1 out]
          n233 = call <vilib>:"Clear Errors.vi"("error in (no error)"=w232) -> ()  [unwired: 6 in, 1 out]
          n234 = while {
            shift-right: [w294] -> w234
            shift-left: w215 -> [w293]
            tunnel: 100000 ("NumberOfBytes") -> [w291]
            tunnel: w229 -> [w289]
            tunnel: [w286] -> w212
            shift-right: [w284] -> w218
            shift-left: w215 -> [w283]
            tunnel: "(41) Execute parse on computer's RAM (faster):" -> [w282]
            i -> [w285]
            stop <- w281 stop-if-true
            n235 = while {
              tunnel: [w303] -> w288
              tunnel: [w302] -> w295
              shift-right: [w300] -> _
              shift-left: 0 ("NumberOfBytes") -> [w301]
              tunnel: w291 -> [w299]
              tunnel: [w297] -> w290
              tunnel: "(36) Round time to 4th decimal place:" -> [w296]
              stop <- w298 stop-if-true
              n236 = call "parse HarpMessage.vi"("Round value"=w296) -> ("HarpDataFrame"=w303:T16, "Packet Found"=w302:bool)  [unwired: 12 in, 1 out]
              n237 = Increment(x=w301) -> (x+1=w300:i32)
              n238 = Equal?(x=w300, y=w299) -> (x = y?=w297:bool)
              n239 = Or(x=w297, y=w302) -> (x .or. y?=w298:bool)
            }
            n240 = Or(x="abort", y=w290) -> (x .or. y?=w281:bool)
            n241 = case shown="True" w295 {
              tunnel: w288 -> [_ w325]
              tunnel: [w306 w312] -> w294
              tunnel: w293 -> [w306 w324]
              tunnel: w289 -> [w305 w319]
              tunnel: w288 -> [_ w323]
              tunnel: [w305 w319] -> w286
              tunnel: w285 -> [_ w318]
              tunnel: [w304 w313] -> w284
              tunnel: w283 -> [w304 w315]
              tunnel: w282 -> [_ w314]
              frame False {
              }
              frame True {
                n242 = local read "For separation, use Tab instead of Comma:"() -> (w309:bool)
                n243 = local read "System (copy)"() -> (w322:bool)
                n244 = Less?(x=w318, y=2000) -> (x < y?=w316:bool)
                n245 = call "create lines.vi"("HarpDataFrame"=w323, "use system decimal point (T)"=w322, "EnableList"="EnableList", "Filter:"="(39) Filter:", "List:"="(40) List:") -> ("Line"=w310:string)  [unwired: 10 in]
                n246 = local read "System"() -> (w308:bool)
                n247 = case shown="True" w316 {
                  tunnel: w325 -> [_ w345]
                  tunnel: w324 -> [w337 w344]
                  tunnel: [w337 w343] -> w312
                  tunnel: w309 -> [_ w339]
                  tunnel: w308 -> [_ w338]
                  frame False {
                  }
                  frame True {
                    n248 = local read "System (copy)"() -> (w342:bool)
                    n249 = call "create metadata.vi"("HarpDataFrame"=w345, "use system decimal point (T)"=w342, "Enum"=enum16{"Find Match", "Reset"}."Find Match") -> ("Line"=w341:string)  [unwired: 11 in, 1 out]
                    n250 = case shown="True" w339 {
                      tunnel: [w347 w350] -> w340
                      tunnel: w341 -> [w347 w349]
                      tunnel: w338 -> [_ w348]
                      frame False {
                      }
                      frame True {
                        n251 = call "comma to tab converter.vi"("System (T: system, F: period)"=w348, "',' string"=w349) -> ("'\\t' string"=w350:string)  [unwired: 13 in]
                      }
                    }
                    n252 = Concatenate Strings(w344, w340) -> (w343:string)
                  }
                }
                n253 = case shown="True" w309 {
                  tunnel: [w326 w329] -> w311
                  tunnel: w310 -> [w326 w328]
                  tunnel: w308 -> [_ w327]
                  frame False {
                  }
                  frame True {
                    n254 = call "comma to tab converter.vi"("System (T: system, F: period)"=w327, "',' string"=w328) -> ("'\\t' string"=w329:string)  [unwired: 13 in]
                  }
                }
                n255 = case shown="True" w314 {
                  tunnel: w319 -> [w332 _]
                  tunnel: w311 -> [w331 w334]
                  tunnel: w315 -> [w330 w336]
                  tunnel: [w330 w335] -> w313
                  frame False {
                    n256 = Write to Text File(file (use dialog)=w332, text=w331) -> (error out=w333:errorcluster)  [unwired: 2 in, 2 out]
                    n257 = call <vilib>:"Clear Errors.vi"("error in (no error)"=w333) -> ()  [unwired: 6 in, 1 out]
                  }
                  frame True {
                    n258 = Concatenate Strings(w336, w334) -> (w335:string)
                  }
                }
              }
            }
          }
          n259 = while {
            tunnel: w242 -> [w370]
            tunnel: [w368] -> w244
            shift-right: [w365] -> _
            shift-left: 0 -> [w366]
            tunnel: w239 -> [w364]
            tunnel: [1.0 ("Creating CSV")] -> w226
            i -> [w360]
            stop <- w353 stop-if-true
            w369 = 8096 ("y")
            # "8KB"
            n260 = call "circular buffer handler.vi"("Enum"=T13."AvailableMemory") -> ("Output"=w362:i32)  [unwired: 12 in, 2 out]
            n261 = Wait (ms)(milliseconds to wait=u32 2) -> ()  [unwired: 1 out]
            n262 = Quotient & Remainder(x=w360, y=10) -> (x-y*floor(x/y)=w358:i32)  [unwired: 1 out]
            n263 = Greater Or Equal?(x=w362, y=w369) -> (x >= y?=w356:bool)
            n264 = Equal To 0?(x=w358) -> (x = 0?=w355:bool)
            n265 = case shown="True" w356 {
              tunnel: w370 -> [w375 w383]
              tunnel: w369 -> [_ w382]
              tunnel: [errorcluster {"status"=FALSE, "code"=0, "source"=""} ("error out") w379] -> w354
              tunnel: [w375 w378] -> w368
              tunnel: [0 w376] -> w367
              frame False {
              }
              frame True {
                n266 = Read from Binary File(10:w382, 11:w383) -> (0:w379:errorcluster, 2:w381:string, 3:w378:refnum<file>)  [unwired: 4 in, 1 out]
                n267 = String To Byte Array(string=w381) -> (unsigned byte array=w377:u8[])
                n268 = Array Size(array=w377) -> (size(s)=w376:i32)
                n269 = call "circular buffer handler.vi"("StreamToWrite"=w377, "Enum"=T13."WriteBytes") -> ()  [unwired: 11 in, 3 out]
              }
            }
            n270 = Add(x=w367, y=w366) -> (x+y=w365:i32)
            n271 = Divide(x=w365, y=w364) -> (x/y=w363:dbl)
            n272 = case shown="True" w355 {
              tunnel: w363 -> [_ w372]
              frame False {
              }
              frame True {
                "Progress:" <- w372
                "File progress:" <- w372
              }
            }
            n273 = local read "abort"() -> (w352:bool)
            n274 = Unbundle By Name(w354) -> ("status"=w351:bool)
            n275 = Or(x=w351, y=w352) -> (x .or. y?=w353:bool)
          }
          n276 = Close File(refnum=w244) -> (error out=w243:errorcluster)  [unwired: 1 in, 1 out]
          n277 = local write "Progress:"(w226) -> ()
          n278 = local write "File progress:"(w226) -> ()
          n279 = call <vilib>:"Clear Errors.vi"("error in (no error)"=w243) -> ()  [unwired: 6 in, 1 out]
          n280 = flat-sequence {
            tunnel: [w246] -> w213
            tunnel: w212 -> [_]
            frame #0 {
              n281 = local read "Tab Control"() -> (w254:T2)
              n282 = local read "abort"() -> (w250:bool)
              n283 = Not(x="don't\nask") -> (.not. x?=w245:bool)
              n284 = Not(x=w250) -> (.not. x?=w249:bool)
              n285 = Equal?(x=w254, y=T9."Create CSV file") -> (x = y?=w252:bool)
              n286 = property on="abort" class="Bool (strict)"("Visible"=FALSE) -> ()  [unwired: 2 in, 2 out]
              n287 = And(x=w249, y=w252) -> (x .and. y?=w251:bool)
              n288 = And(x=w245, y=w251) -> (x .and. y?=w246:bool)
            }
          }
          n289 = Write to Text File(file (use dialog)=w212, text=w218) -> (refnum out=w221:refnum<file>, error out=w220:errorcluster)  [unwired: 2 in, 1 out]
          n290 = call <vilib>:"Clear Errors.vi"("error in (no error)"=w220) -> ("error out"=w219:errorcluster)  [unwired: 6 in]
          n291 = Close File(refnum=w221, error in=w219) -> (path=w227:path, error out=w228:errorcluster)
          n292 = Write to Text File(file (use dialog)=w233, text=w234) -> (refnum out=w224:refnum<file>, error out=w236:errorcluster)  [unwired: 2 in, 1 out]
          n293 = call <vilib>:"Clear Errors.vi"("error in (no error)"=w228) -> ()  [unwired: 6 in, 1 out]
          n294 = case shown="False" w213 {
            tunnel: w227 -> [_ w270]
            tunnel: [TRUE FALSE] -> w222
            tunnel: [w255 w266] -> w217
            frame False {
              n295 = Tick Count (ms)() -> (millisecond timer value=w255:u32)
            }
            frame True {
              n296 = Strip Path(path=w270) -> (name=w260:string)  [unwired: 1 out]
              n297 = Concatenate Strings("File \"" ("message"), w260, "\" was created." ("string")) -> (w258:string)
              n298 = property on="dummy" class="DigNum (strict)"("Caption.Text"="") -> ()  [unwired: 2 in, 2 out]
              n299 = call <vilib>:"Three Button Dialog.vi"("Allow user to close window? (TRUE)"=FALSE, "Justify Message (Left)"=enum16{"Left", "Center", "Right"}."Center", "Right Button Text (\"Cancel\")"="Open file location" ("F button name (\"Cancel\")"), "Center Button Text (\"No\")"="Open file" ("F button name (\"Cancel\")"), "Left Button Text (\"Yes\")"="Done" ("T button name (\"OK\")"), "message"=w258) -> ("Which Button?"=w269:T17)  [unwired: 5 in]
              n300 = case shown="\"Right Button\"" w269 {
                tunnel: w270 -> [w272 w276 _]
                frame "Right Button" {
                  n301 = Strip Path(path=w272) -> (stripped path=w271:path)  [unwired: 1 out]
                  n302 = Format Into String(format string="cmd /c explorer.exe \"%s\"", w271) -> (resulting string=w275:string)  [unwired: 2 in, 1 out]
                  n303 = call <vilib>:"System Exec.vi"("run minimized? (F)"=TRUE, "command line"=w275) -> ()  [unwired: 6 in, 4 out]
                }
                frame "Center Button" {
                  n304 = Format Into String(format string="cmd /c explorer.exe \"%s\"", w276) -> (resulting string=w279:string)  [unwired: 2 in, 1 out]
                  n305 = call <vilib>:"System Exec.vi"("run minimized? (F)"=TRUE, "command line"=w279) -> ()  [unwired: 6 in, 4 out]
                }
                frame "Left Button", Default {
                }
              }
              n306 = Tick Count (ms)() -> (millisecond timer value=w266:u32)
            }
          }
          n307 = Close File(refnum=w224, error in=w236) -> (error out=w235:errorcluster)  [unwired: 1 out]
          n308 = call <vilib>:"Clear Errors.vi"("error in (no error)"=w235) -> ()  [unwired: 6 in, 1 out]
        }
        frame Error {
          w385 = TRUE ("Error Ctrl")
          n309 = local read "Tab Control"() -> (w393:T2)
          n310 = Strip Path(path=w390) -> (name=w388:string)  [unwired: 1 out]
          n311 = Concatenate Strings(w387, w388, "\r\n") -> (w386:string)
          n312 = Equal?(x=w393, y=T9."Create CSV file") -> (x = y?=w391:bool)
          n313 = case shown="True" w391 {
            tunnel: w397 -> [_ w398]
            frame False {
            }
            frame True {
              n314 = case shown="Error" w398 {
                frame No Error {
                }
                frame Error {
                  w400 = "Not able to open the file." ("message")
                  n315 = local read "don't\nask"() -> (w399:bool)
                  n316 = local write "error"(w400) -> ()
                  n317 = case shown="False" w399 {
                    tunnel: w400 -> [w401 _]
                    frame False {
                      n318 = One Button Dialog(message=w401) -> ()  [unwired: 1 in, 1 out]
                    }
                    frame True {
                    }
                  }
                }
              }
            }
          }
          n319 = case shown="False" FALSE {
            tunnel: errorcluster {"status"=FALSE, "code"=0, "source"=""} ("error IO") -> [w403 _]
            tunnel: errorcluster {"status"=FALSE, "code"=0, "source"=""} ("error IO") -> [w402 _]
            frame False {
              n320 = case shown="No Error" w403 {
                tunnel: w402 -> [w404 _]
                frame No Error {
                  n321 = case shown="No Error" w404 {
                    frame No Error {
                    }
                    frame Error {
                      n322 = local read "don't\nask"() -> (w405:bool)
                      n323 = case shown="False" w405 {
                        frame False {
                          w406 = "Not able to create the .csv file.\nDo you have privileges to create the file?\nThe file is open?" ("message")
                          n324 = local write "error"(w406) -> ()
                          n325 = One Button Dialog(message=w406) -> ()  [unwired: 1 in, 1 out]
                        }
                        frame True {
                        }
                      }
                    }
                  }
                }
                frame Error {
                }
              }
            }
            frame True {
            }
          }
          n326 = local write "Error Ctrl"(w385) -> ()
        }
      }
      n327 = Subtract(x=w189, y=w187) -> (x-y=→"conversion\ntime":u32)
    }
    n328 = flat-sequence {
      tunnel: w83 -> [w161]
      tunnel: [w157] -> w81
      tunnel: w75 -> [w149]
      frame #0 {
        w141 = T12."Save error" ("option")
        n329 = local read "abort"() -> (w160:bool)
        n330 = local read "Error Ctrl"() -> (w142:bool)
        n331 = local read "don't\nask"() -> (w138:bool)
        n332 = local read "Tab Control"() -> (w148:T2)
        n333 = local write "Convert 2"(FALSE ("Convert")) -> ()
        n334 = property on="abort" class="Bool (strict)"("Visible"=FALSE) -> ()  [unwired: 2 in, 2 out]
        n335 = local write "Convert"(FALSE ("Convert")) -> ()
        n336 = Not(x=w160) -> (.not. x?=w159:bool)
        n337 = And(x=w159, y=w161) -> (x .and. y?=w153:bool)
        n338 = Select(t=T12."Unfreeze" ("option"), s=w153, f=w141) -> (s? t:f=w140:T12)
        n339 = Select(t=w141, s=w142, f=w140) -> (s? t:f=w139:T12)
        n340 = Equal?(x=w148, y=T9."Create CSV file") -> (x = y?=w146:bool)
        n341 = Not(x=w138) -> (.not. x?=w156:bool)
        n342 = local read "Error Ctrl"() -> (w145:bool)
        n343 = And(x=w153, y=w156) -> (x .and. y?=w157:bool)
        n344 = Select(t=FALSE, s=w146, f=w145) -> (s? t:f=w143:bool)
        n345 = Select(t=w149, s=w143, f="error") -> (s? t:f=w150:string)
        n346 = case shown="True" w138 {
          tunnel: w150 -> [_ w163]
          tunnel: w139 -> [_ w162]
          frame False {
          }
          frame True {
            n347 = call "external cmd - main.vi"("error"=w163, "option"=w162) -> ()  [unwired: 10 in, 4 out]
          }
        }
      }
    }
    n348 = case shown="True" w81 {
      tunnel: w75 -> [_ w176]
      tunnel: [_ w169] -> w82
      frame False {
        n349 = local write "don't\nask"(FALSE ("don't\nopen")) -> ()
      }
      frame True {
        n350 = local read "Error Ctrl"() -> (w175:bool)
        n351 = case shown="True" w175 {
          tunnel: w176 -> [_ w183]
          tunnel: "Files were created.\nOpen location folder?" ("message") -> [w181 w182]
          tunnel: [w181 w182] -> w170
          frame False {
          }
          frame True {
            n352 = One Button Dialog(message=w183) -> ()  [unwired: 1 in, 1 out]
          }
        }
        n353 = local write "Overall progress:"(1.0 ("Overall progress:")) -> ()
        n354 = Two Button Dialog(message=w170, 1:"Yes" ("F button name (\"Cancel\")"), 2:"No" ("T button name (\"OK\")")) -> (T button?=w169:bool)
        n355 = case shown="False" w169 {
          frame False {
            n356 = local read "Path (folder)"() -> (w177:path)
            n357 = Format Into String(format string="cmd /c explorer.exe \"%s\"", w177) -> (resulting string=w180:string)  [unwired: 2 in, 1 out]
            n358 = call <vilib>:"System Exec.vi"("run minimized? (F)"=TRUE, "command line"=w180) -> ()  [unwired: 6 in, 4 out]
          }
          frame True {
          }
        }
      }
    }
    n359 = flat-sequence {
      tunnel: w82 -> [_]
      frame #0 {
        n360 = local write "Overall progress:"(1.0 ("Overall progress:")) -> ()
        n361 = local write "File progress:"(1.0 ("File progress:")) -> ()
        n362 = property on="dummy" class="DigNum (strict)"("Caption.Text"="") -> ()  [unwired: 2 in, 2 out]
        n363 = property on="Tab Control" class="TabCtl (strict)"("DisabledEnum"=T10."Enabled" ("Disabled")) -> ()  [unwired: 2 in, 2 out]
      }
    }
  }
  n364 = while {
    tunnel: w4 -> [_]
    stop <- FALSE stop-if-true
    n365 = while {
      stop <- FALSE ("stop") stop-if-true
      n366 = Wait (ms)(milliseconds to wait=u32 20) -> ()  [unwired: 1 out]
      n367 = call "external cmd - main.vi"("option"=T6."Open files") -> ()  [unwired: 11 in, 4 out]
    }
    n368 = while {
      stop <- FALSE stop-if-true
      n369 = Wait (ms)(milliseconds to wait=u32 10) -> ()  [unwired: 1 out]
      n370 = call "external cmd - main.vi"("option"=T6."Get command") -> ("address"=w587:u8, "content"=w586:string, "is true"=w585:bool, "cmd available"=w588:bool)  [unwired: 11 in]
      n371 = case shown="True" w588 {
        tunnel: w587 -> [_ w591]
        tunnel: w586 -> [_ w593]
        tunnel: w585 -> [_ w592]
        frame False {
        }
        frame True {
          n372 = case shown="210" w591 {
            tunnel: w593 -> [_ w625 w626 _ _ w630 w631 _ _ _ _ _ _ _ _ _ w643 w644 _ w646 w648 _ w652 _ _ _ _ _]
            tunnel: w592 -> [_ _ _ w628 w629 _ _ w632 w633 w634 w635 w636 w637 w638 w639 w640 _ _ w645 _ _ w650 _ w655 w661 w668 w669 w670]
            frame 0, Default {
            }
            frame 1 {
              n373 = String To Path(string=w625) -> (path=w624:path)
              n374 = local write "Path (file)"(w624) -> ()
            }
            frame 10 {
              n375 = String To Path(string=w626) -> (path=w627:path)
              n376 = local write "Path (folder)"(w627) -> ()
            }
            frame 11 {
              n377 = local write "(11) Overwrite .csv files:"(w628) -> ()
            }
            frame 12 {
              n378 = local write "(12) Include subfolders:"(w629) -> ()
            }
            frame 13 {
              n379 = local write "(13) File extension:"(w630) -> ()
            }
            frame 14 {
              n380 = local write "(14) Match pattern:"(w631) -> ()
            }
            frame 30 {
              n381 = local write "(30) Create \"read me\" information file:"(w632) -> ()
            }
            frame 31 {
              n382 = local write "System"(w633) -> ()
            }
            frame 32 {
              n383 = local write "(32) Read"(w634) -> ()
            }
            frame 33 {
              n384 = local write "(33) Write"(w635) -> ()
            }
            frame 34 {
              n385 = local write "(34) Event"(w636) -> ()
            }
            frame 35 {
              n386 = local write "(35) Save only if no error:"(w637) -> ()
            }
            frame 36 {
              n387 = local write "(36) Round time to 4th decimal place:"(w638) -> ()
            }
            frame 37 {
              n388 = local write "(37) Insert Bit Demux Elements at the end:"(w639) -> ()
            }
            frame 38 {
              n389 = local write "(38) Include entire information:"(w640) -> ()
            }
            frame 39 {
              n390 = Decimal String To Number(string=w643, default (0L)=u16 0 ("default (0 I32)")) -> (number=w641:u16)  [unwired: 1 in, 1 out]
              n391 = local write "(39) Filter:"(w641) -> ()
            }
            frame 40 {
              n392 = local write "(40) List:"(w644) -> ()
            }
            frame 41 {
              n393 = local write "(41) Execute parse on computer's RAM (faster):"(w645) -> ()
            }
            frame 60 {
              n394 = String To Path(string=w646) -> (path=w647:path)
              n395 = local write "harp .bin"(w647) -> ()
            }
            frame 61 {
              n396 = String To Path(string=w648) -> (path=w649:path)
              n397 = local write "cam .csv"(w649) -> ()
            }
            frame 62 {
              n398 = local write "(62) Use Harp converted .csv file\nto timestamp the file:"(w650) -> ()
            }
            frame 64 {
              n399 = Decimal String To Number(string=w652, default (0L)=u16 0 ("default (0 I32)")) -> (number=w651:u16)  [unwired: 1 in, 1 out]
              n400 = local write "(64) Register Address:"(w651) -> ()
            }
            frame 200 {
              n401 = flat-sequence {
                tunnel: [w659] -> w654
                tunnel: w655 -> [w659]
                frame #0 {
                  n402 = local write "don't\nask"(TRUE ("don't\nopen")) -> ()
                  n403 = local write "Tab Control"(T2."Create CSV file" ("Tab Control")) -> ()
                  n404 = call "external cmd - main.vi"("option"=T6."Freeze") -> ()  [unwired: 11 in, 4 out]
                  n405 = Wait (ms)(milliseconds to wait=u32 100) -> ()  [unwired: 1 out]
                }
              }
              n406 = local write "Convert"(w654) -> ()
            }
            frame 205 {
              n407 = flat-sequence {
                tunnel: [w666] -> w662
                tunnel: w661 -> [w666]
                frame #0 {
                  n408 = local write "don't\nask"(TRUE ("don't\nopen")) -> ()
                  n409 = local write "Tab Control"(T2."Create multiple CSV files" ("Tab Control")) -> ()
                  n410 = call "external cmd - main.vi"("option"=T6."Freeze") -> ()  [unwired: 11 in, 4 out]
                  n411 = Wait (ms)(milliseconds to wait=u32 100) -> ()  [unwired: 1 out]
                }
              }
              n412 = local write "Convert 2"(w662) -> ()
            }
            frame 210 {
              n413 = local write "Minimize"(w668) -> ()
            }
            frame 211 {
              n414 = local write "Quit"(w669) -> ()
            }
            frame 215 {
              n415 = flat-sequence {
                tunnel: [w673] -> w671
                tunnel: w670 -> [w673]
                frame #0 {
                  n416 = local write "don't\nask"(TRUE ("don't\nopen")) -> ()
                  n417 = call "external cmd - main.vi"("option"=T6."Freeze") -> ()  [unwired: 11 in, 4 out]
                }
              }
              n418 = local write "Convert 3"(w671) -> ()
            }
          }
          n419 = stacked-sequence {
            tunnel: w591 -> [w594 w614]
            frame #0 {
              n420 = In Range and Coerce(upper limit=u8 9, x=w594, lower limit=u8 1) -> (In Range?=w604:bool)  [unwired: 1 out]
              n421 = In Range and Coerce(upper limit=u8 29, x=w594, lower limit=u8 10) -> (In Range?=w603:bool)  [unwired: 1 out]
              n422 = In Range and Coerce(upper limit=u8 49, x=w594, lower limit=u8 30) -> (In Range?=w598:bool)  [unwired: 1 out]
              n423 = In Range and Coerce(upper limit=u8 69, x=w594, lower limit=u8 60) -> (In Range?=w597:bool)  [unwired: 1 out]
              n424 = case shown="True" w604 {
                frame False {
                }
                frame True {
                  n425 = local write "Tab Control"(T2."Create CSV file" ("Tab Control")) -> ()
                }
              }
              n426 = case shown="True" w603 {
                frame False {
                }
                frame True {
                  n427 = local write "Tab Control"(T2."Create multiple CSV files" ("Tab Control")) -> ()
                }
              }
              n428 = case shown="True" w598 {
                frame False {
                }
                frame True {
                  n429 = local write "Tab Control"(T2."Options" ("Tab Control")) -> ()
                }
              }
              n430 = case shown="True" w597 {
                frame False {
                }
                frame True {
                  n431 = local write "Tab Control"(T2."Video Synchronization" ("Tab Control")) -> ()
                }
              }
            }
            frame #1 {
              n432 = Equal?(x=w614, y=u8 200) -> (x = y?=w618:bool)
              n433 = Equal?(x=w614, y=u8 205) -> (x = y?=w613:bool)
              n434 = Equal?(x=w614, y=u8 211) -> (x = y?=w612:bool)
              n435 = Equal?(x=w614, y=u8 215) -> (x = y?=w611:bool)
              n436 = case shown="True" w618 {
                frame False {
                }
                frame True {
                  n437 = local write "Tab Control"(T2."Create CSV file" ("Tab Control")) -> ()
                }
              }
              n438 = case shown="True" w613 {
                frame False {
                }
                frame True {
                  n439 = local write "Tab Control"(T2."Create multiple CSV files" ("Tab Control")) -> ()
                }
              }
              n440 = case shown="True" w612 {
                frame False {
                }
                frame True {
                  n441 = local write "Tab Control"(T2."Options" ("Tab Control")) -> ()
                }
              }
              n442 = case shown="True" w611 {
                frame False {
                }
                frame True {
                  n443 = local write "Tab Control"(T2."Video Synchronization" ("Tab Control")) -> ()
                }
              }
            }
          }
        }
      }
    }
  }
